vi "Limelight_Read.vi"   [LabVIEW 2019]
uses:
  <vilib>/Rock Robotics/Network Tables/NT Read Number.vi
  Sensor_Values.vi
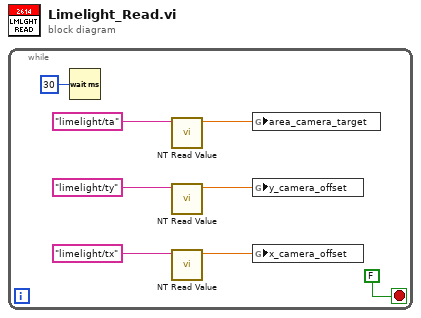
[diagram p0: block diagram]
diagram:
  n1 = while {
    stop <- FALSE stop-if-true
    n2 = Wait (ms)(milliseconds to wait=u32 30) -> ()  [unwired: 1 out]
    n3 = call-poly <vilib>:"NT Read Value.vi"("Name"="limelight/ta") -> ("Numeric"=w1:dbl)  [unwired: 9 in, 1 out]
    n4 = call-poly <vilib>:"NT Read Value.vi"("Name"="limelight/ty") -> ("Numeric"=w4:dbl)  [unwired: 9 in, 1 out]
    n5 = call-poly <vilib>:"NT Read Value.vi"("Name"="limelight/tx") -> ("Numeric"=w3:dbl)  [unwired: 9 in, 1 out]
    n6 = global write "Sensor_Values.vi" "area_camera_target"(w1) -> ()
    n7 = global write "Sensor_Values.vi" "y_camera_offset"(w4) -> ()
    n8 = global write "Sensor_Values.vi" "x_camera_offset"(w3) -> ()
  }
